vi "PPL_SIM_SIM_INIT.vi"(8 "error in (no error)":errorcluster, 11 "Initial Robot Position":T1 {"ROTATION"."SIN" format="%13.4f"; "ROTATION"."COS" format="%13.4f"; "ROTATION"."VALUE" format="%13.4f"; "TRANSLATION"."Y" format="%14.3f"; "TRANSLATION"."X" format="%14.3f"}) -> (0 "error out":errorcluster)   [LabVIEW 2019]
uses:
  <vilib>/Rock Robotics/SystemInterfaces/DIO/FPGA_DIOPWMChannel.ctl
  <vilib>/Rock Robotics/SystemInterfaces/DIO/FPGA_DIOChannel.ctl
  <vilib>/Rock Robotics/WPI/ThirdParty/JAS_Junk/TrajLib/Trajectory_Library.lvlib
  PPL_SIM_SIM_Globals.vi
  <vilib>/Rock Robotics/WPI/ThirdParty/JAS_Junk/TrajLib/TypeDef/TRANSLATION2D.ctl
  <vilib>/Rock Robotics/WPI/ThirdParty/JAS_Junk/TrajLib/TypeDef/ROTATION2D.ctl
  <vilib>/Rock Robotics/WPI/ThirdParty/JAS_Junk/TrajLib/TypeDef/POSE2D.ctl
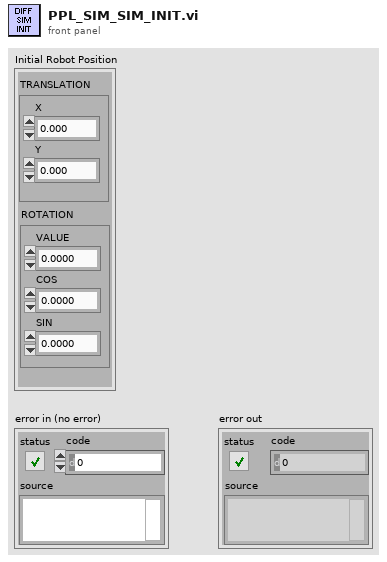
[diagram p1: front panel]
types:
  T1 = typedef "Trajectory_Library.lvlib/POSE2D.ctl" = cluster{"TRANSLATION":T2, "ROTATION":T3}
  T2 = typedef "Trajectory_Library.lvlib/TRANSLATION2D.ctl" = cluster{"X":dbl, "Y":dbl}
  T3 = typedef "Trajectory_Library.lvlib/ROTATION2D.ctl" = cluster{"VALUE":dbl, "COS":dbl, "SIN":dbl}
  T4 = typedef "FPGA_DIOChannel.ctl" = enum8{"DIO 0", "DIO 1", "DIO 2", "DIO 3", "DIO 4", "DIO 5", "DIO 6", "DIO 7", "DIO 8", "DIO 9", "DIO MXP 0", "DIO MXP 1", "DIO MXP 2", "DIO MXP 3", "DIO MXP 4", "DIO MXP 5", "DIO MXP 6", "DIO MXP 7", "DIO MXP 8", "DIO MXP 9", "DIO MXP 10", "DIO MXP 11", "DIO MXP 12", "DIO MXP 13", "DIO MXP 14", "DIO MXP 15", "SPI Port CS1", "SPI Port CS2", "SPI Port CS3", "SPI Port MISO", "SPI Port MOSI", "Invalid"}
  T5 = typedef "FPGA_DIOPWMChannel.ctl" = enum8{"PWM 0", "PWM 1", "PWM 2", "PWM 3", "PWM 4", "PWM 5", "PWM 6", "PWM 7", "PWM 8", "PWM 9", "PWM MXP 0", "PWM MXP 1", "PWM MXP 2", "PWM MXP 3", "PWM MXP 4", "PWM MXP 5", "PWM MXP 6", "PWM MXP 7", "PWM MXP 8", "PWM MXP 9", "Invalid"}
  T6 = enum32{"Invalid", "Standard", "Closed", "Hidden", "Minimized", "Maximized"}
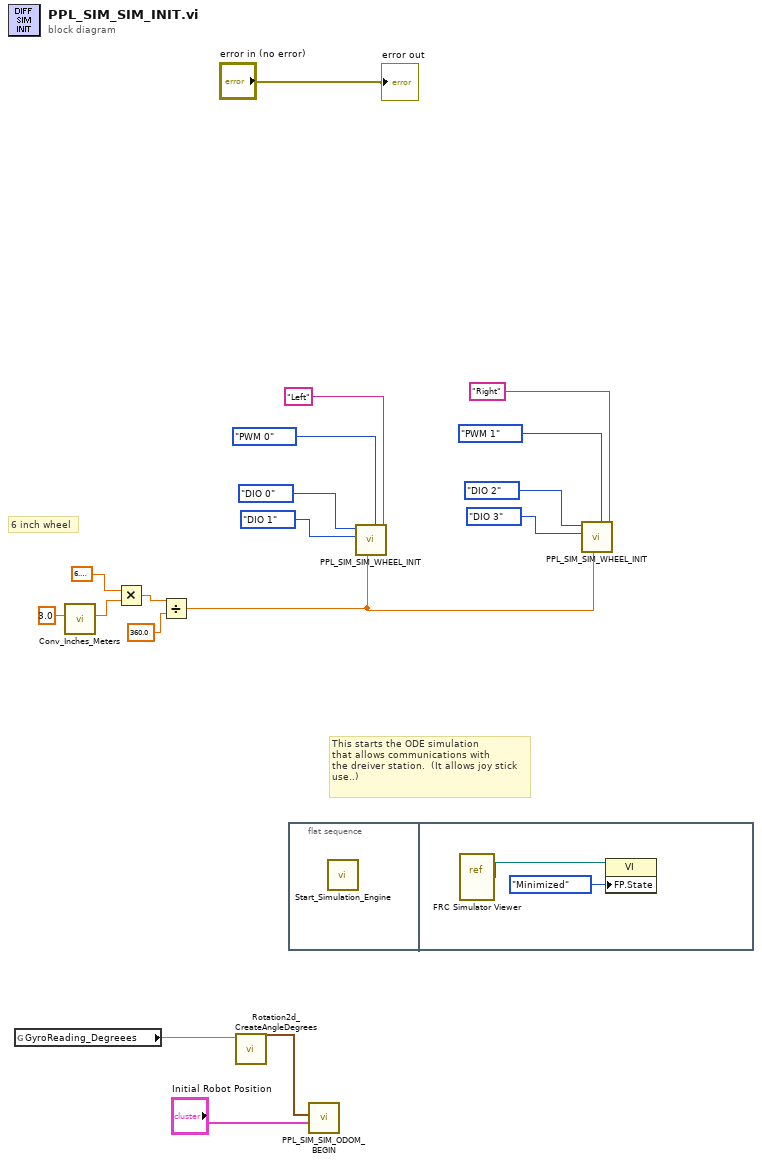
[diagram p0: block diagram]
diagram:
  # "This starts the ODE simulation\nthat allows communications with\nthe dreiver station.  (It allows joy stick\nuse..)"
  # "6 inch wheel"
  n1 = global read "PPL_SIM_SIM_Globals.vi" "GyroReading_Degreees"() -> (w4:dbl)
  n2 = call <vilib>:"Conv_Inches_Meters.vi"("INCH"=3.0) -> ("Meters"=w16:dbl)  [unwired: 10 in]
  n3 = Multiply(x=6.283185307179586, y=w16) -> (x*y=w7:dbl)
  n4 = Divide(x=w7, y=360.0) -> (x/y=w18:dbl)
  n5 = call <vilib>:"Rotation2d_CreateAngleDegrees.vi"("Angle_Degrees"=w4) -> ("ROTATION"=w3:T3)  [unwired: 10 in]
  n6 = flat-sequence {
    frame #0 {
      n7 = call <vilib>:"Start_Simulation_Engine.vi"() -> ()  [unwired: 15 in, 1 out]
    }
    frame #1 {
      n8 = vi-ref <vilib>:"FRC Simulator Viewer.vi"() -> (w20:refnum<vi>)
      n9 = property class="VI"(reference=w20, "FP.State"=T6."Minimized" ("Front Panel Window:State")) -> ()  [unwired: 1 in, 2 out]
    }
  }
  n10 = call "PPL_SIM_SIM_ODOM_BEGIN.vi"("Initial Pose"="Initial Robot Position", "Initial Gyro Angle"=w3) -> ()  [unwired: 9 in, 1 out]
  n11 = call "PPL_SIM_SIM_WHEEL_INIT.vi"("Side"="Left", "Drive PWM Channel"=FPGA_DIOPWMChannel."PWM 0", "DriveDistPerCount"=w18, "Drive B Channel"=FPGA_DIOChannel."DIO 1", "Drive A channel"=FPGA_DIOChannel."DIO 0") -> ()  [unwired: 7 in]
  n12 = call "PPL_SIM_SIM_WHEEL_INIT.vi"("Side"="Right", "Drive PWM Channel"=FPGA_DIOPWMChannel."PWM 1", "DriveDistPerCount"=w18, "Drive B Channel"=FPGA_DIOChannel."DIO 3", "Drive A channel"=FPGA_DIOChannel."DIO 2") -> ()  [unwired: 7 in]
  "error out" <- "error in (no error)"
